vi "Load New AVI.vi"(8 "error in (no error)":errorcluster, 11 "AVI Path":path) -> (0 "error out":errorcluster, 3 "Image Array":T1[](array[typedef]))   [LabVIEW 2013]
uses:
  <vilib>/vision/Image Controls.llb/IMAQ Image.ctl
  <vilib>/vision/NI_Vision_Development_Module.lvlib
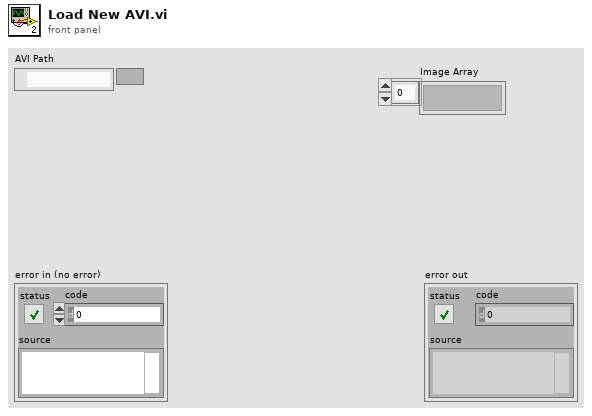
[diagram p1: front panel]
types:
  T1 = typedef "IMAQ Image.ctl" = refnum<image>
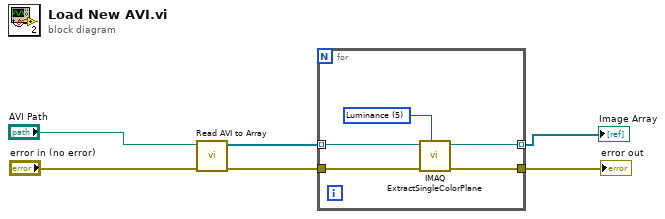
[diagram p0: block diagram]
diagram:
  n1 = call "Read AVI to Array.vi"("Error in (no error)"="error in (no error)", "AVI Path"="AVI Path") -> ("Error out"=w3:errorcluster, "Image Array"=w4:T1[])  [unwired: 7 in, 1 out]
  n2 = for {
    tunnel: w4 -> [w10] mode=indexing
    tunnel: w3 -> [w11]
    tunnel: [w8] -> w1 mode=indexing
    tunnel: [w7] -> w2
    w9 = 5 items=["Red", "Green", "Blue", "Hue", "Saturation", "Luminance", "Value", "Intensity"] ("Color Plane")
    n3 = call "IMAQ ExtractSingleColorPlane"("Color Plane"=w9, "error in (no error)"=w11, "Image Src"=w10) -> ("error out"=w7:errorcluster, "Image Dst Out"=w8:T1)  [unwired: 7 in]
  }
  "Image Array" <- w1
  "error out" <- w2
